vi "Function.vi"(8 "error in (no error)":errorcluster, 10 "Value":i32, 11 "Two Terminal in":refnum<class "Invert_I32.lvclass">) -> (0 "error out":errorcluster, 2 "Result":i32, 3 "Two Terminal out":refnum<class "Invert_I32.lvclass">)   [LabVIEW 2021, in "Invert_I32.lvclass"]
uses:
  Invert_I32.lvclass
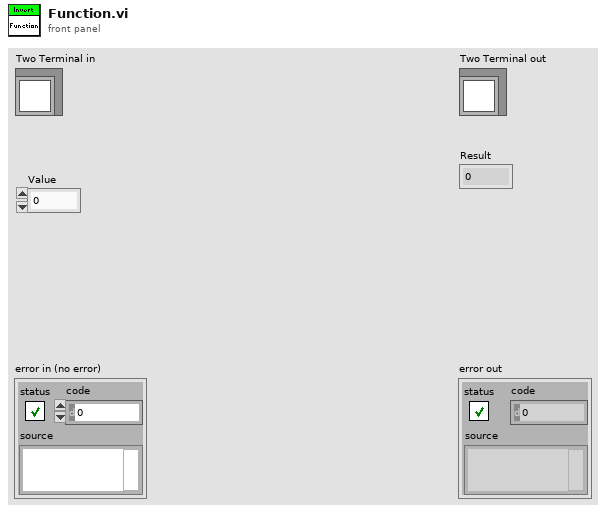
[diagram p1: front panel]
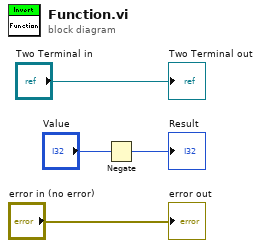
[diagram p0: block diagram]
diagram:
  n1 = Negate(x="Value") -> (-x=→"Result":i32)
  "error out" <- "error in (no error)"
  "Two Terminal out" <- "Two Terminal in"
